vi "Read String Data.vi"(11 "Caller Test Harness in":refnum<class "Caller Test Harness.lvclass">) -> (2 "String Data":string)   [LabVIEW 2020, in "Caller Test Harness.lvlib" / "Caller Test Harness.lvclass"]
uses:
  Caller Test Harness.lvclass
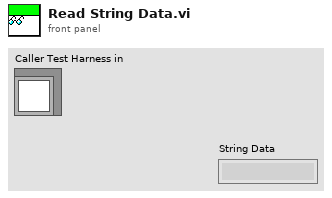
[diagram p1: front panel]
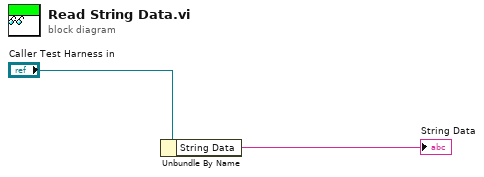
[diagram p0: block diagram]
diagram:
  n1 = Unbundle By Name("Caller Test Harness in") -> ("String Data"=→"String Data":string)
